vi "DFT_Determine If Show UI.vi"(11 "Data":T1={"First Time"=FALSE, "Show Results Window"=FALSE, "Show Results Window Clicked"=FALSE, "Window"=1, "overlap"=50, "Block Duration"=0.1, "Averaging parameters"={"averaging mode"=enum."No averaging", "weighting mode"=enum."Exponential", "number of averages"=10}, "buffer out"=refnum, "Avg Spectra"=refnum, "Spectra UI"=refnum} {"Averaging parameters"."number of averages" min=1; "Window" items=["Rectangle"=0, "Hanning"=1, "Hamming"=2, "Blackman-Harris"=3, "Exact Blackman"=4, "Blackman"=5, "Flat Top"=6, "4 Term B-Harris "=7, "7 Term B-Harris"=8, "Low Sidelobe"=9, "Blackman Nuttall"=11, "Triangle"=30, "Bartlett-Hanning"=31, "Bohman"=32, "Parzen"=33, "Welch"=34, "Kaiser"=60, "Dolph-Chebyshev"=61, "Gaussian"=62]}) -> (2 "Show window":bool, 3 "Data out":T1={"First Time"=FALSE, "Show Results Window"=FALSE, "Show Results Window Clicked"=FALSE, "Window"=1, "overlap"=50, "Block Duration"=0.1, "Averaging parameters"={"averaging mode"=enum."No averaging", "weighting mode"=enum."Exponential", "number of averages"=10}, "buffer out"=refnum, "Avg Spectra"=refnum, "Spectra UI"=refnum} {"Averaging parameters"."number of averages" min=1; "Window" items=["Rectangle"=0, "Hanning"=1, "Hamming"=2, "Blackman-Harris"=3, "Exact Blackman"=4, "Blackman"=5, "Flat Top"=6, "4 Term B-Harris "=7, "7 Term B-Harris"=8, "Low Sidelobe"=9, "Blackman Nuttall"=11, "Triangle"=30, "Bartlett-Hanning"=31, "Bohman"=32, "Parzen"=33, "Welch"=34, "Kaiser"=60, "Dolph-Chebyshev"=61, "Gaussian"=62]})   [LabVIEW 2024, in "DFT_Spectra.lvlib" / "DFT_Spectra.lvclass"]
uses:
  DFT_Spectra.lvclass
  DFT_Spectra Data.ctl
  <vilib>/Analysis/4window.llb/windowTd.ctl
  <vilib>/addons/_NISVFA/_Shared subVIs/Data Objects/Waveforms (DBL)/Waveforms (N Ch).lvclass
  <vilib>/addons/_NISVFA/_Shared subVIs/Data Objects/Data/Data.lvclass
  <vilib>/Analysis/NI_AALPro.lvlib
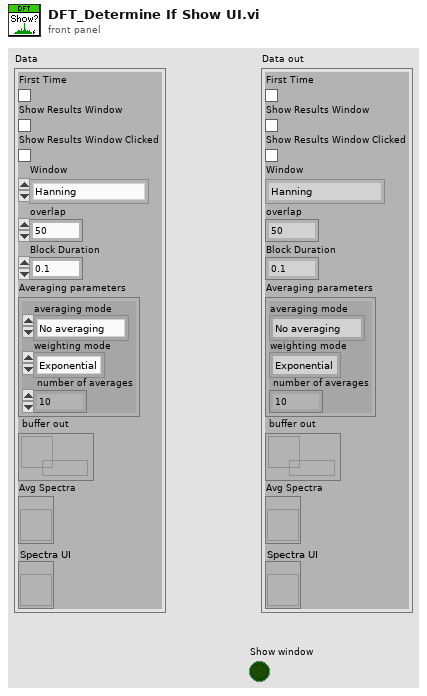
[diagram p1: front panel]
types:
  T1 = typedef "DFT_Spectra.lvlib/DFT_Spectra.lvclass/DFT_Spectra Data.ctl" = cluster{"First Time":bool, "Show Results Window":bool, "Show Results Window Clicked":bool, "Window":T2, "overlap":i32, "Block Duration":dbl, "Averaging parameters":cluster{"averaging mode":enum16{"No averaging", "Vector averaging", "RMS averaging", "Peak hold"}, "weighting mode":enum16{"Linear", "Exponential"}, "number of averages":u32}, "buffer out":refnum<data-value>, "Avg Spectra":refnum<vi>, "Spectra UI":refnum<vi>}
  T2 = typedef "NI_AALPro.lvlib/windowTd.ctl" = u32
  T3 = enum32{"Invalid", "Standard", "Closed", "Hidden", "Minimized", "Maximized"}
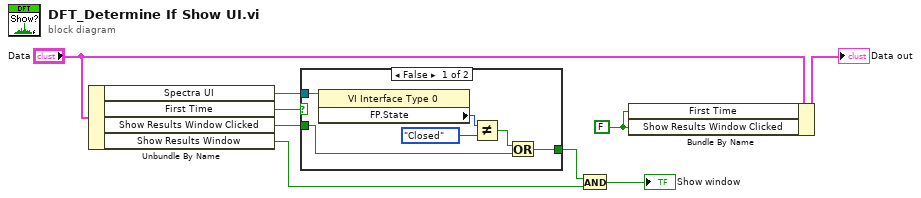
[diagram p0: block diagram]
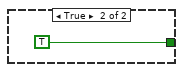
[diagram p2: hidden frame]
diagram:
  w3 = FALSE ("Show Spectrogram Window Button Clicked")
  n1 = Unbundle By Name("Data") -> ("Spectra UI"=w8:refnum<vi>, "First Time"=w2:bool, "Show Results Window Clicked"=w1:bool, "Show Results Window"=w6:bool)
  n2 = case shown="False" w2 {
    tunnel: w8 -> [w15 _]
    tunnel: [w10 TRUE] -> w7
    tunnel: w1 -> [w12 _]
    frame False {
      n3 = property class="VI Interface Type 0"(reference=w15) -> ("FP.State"=w14:T3)  [unwired: 1 in, 2 out]
      n4 = Not Equal?(x=w14, y=T3."Closed" ("Front Panel Window:State")) -> (x != y?=w11:bool)
      n5 = Or(x=w11, y=w12) -> (x .or. y?=w10:bool)
    }
    frame True {
    }
  }
  n6 = And(x=w7, y=w6) -> (x .and. y?=→"Show window":bool)
  n7 = Bundle By Name(cluster="Data", "First Time"=w3, "Show Results Window Clicked"=w3) -> (→"Data out":T1)
